vi "Match Axis NEW (SubVI).vi"(0 "Axis ID":string, 7 "input string":string, 9 "Visa name in":refnum<visa-resource-name>, 11 "error in":errorcluster) -> (2 "Good\nto read!":bool, 4 "out number":dbl, 8 "out string":string, 10 "Visa name out":refnum<visa-resource-name>, 13 "status":bool, 15 "error out":errorcluster)   [LabVIEW 2013]
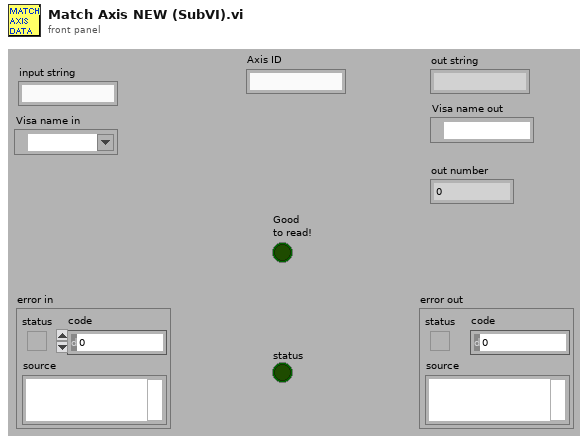
[diagram p1: front panel]
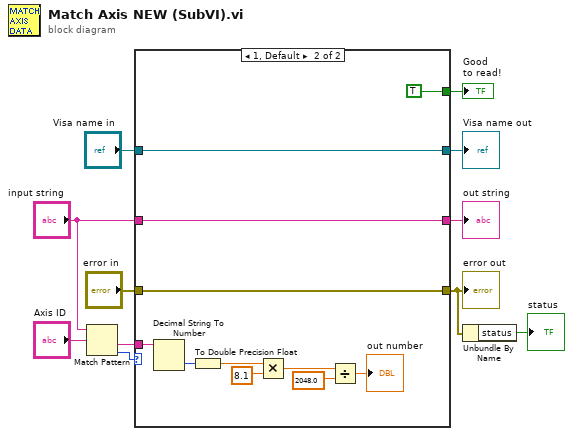
[diagram p0: block diagram]
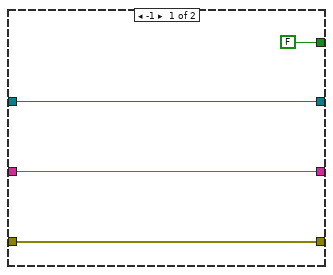
[diagram p2: hidden frame]
diagram:
  n1 = Match Pattern(string="input string", regular expression="Axis ID") -> (after substring=w8:string, offset past match=w7:i32)  [unwired: 3 out]
  n2 = case shown="1, Default" w7 {
    tunnel: [w15 w17] -> w5
    tunnel: w8 -> [_ w23]
    tunnel: "error in" -> [w15 w17]
    tunnel: "Visa name in" -> [w14 w22]
    tunnel: [w14 w22] -> w11
    tunnel: [w13 w20] -> w2
    tunnel: "input string" -> [w13 w20]
    tunnel: [FALSE ("status") TRUE ("status")] -> w1
    frame -1 {
    }
    frame 1, Default {
      n3 = Decimal String To Number(string=w23) -> (number=w26:i32)  [unwired: 3 out]
      n4 = To Double Precision Float(number=w26) -> (double precision float=w21:dbl)
      n5 = Multiply(x=w21, y=8.1) -> (x*y=w25:dbl)
      n6 = Divide(x=w25, y=2048.0) -> (x/y=→"out number":dbl)
    }
  }
  "Visa name out" <- w11
  "error out" <- w5
  "out string" <- w2
  "Good\nto read!" <- w1
  n7 = Unbundle By Name(w5) -> ("status"=→"status":bool)
